vi "401_Sort 2 Column Array By First Column.vi"(1 "Data_Table":string[][](array[string])) -> (0 "Array":string[][](array[string]))   [LabVIEW 2015]
doc: "This vi sorts a two-column array in reference to its first column."
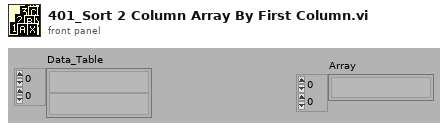
[diagram p1: front panel]
types:
  T1 = cluster{string, string, string, string, string, string, string}[]
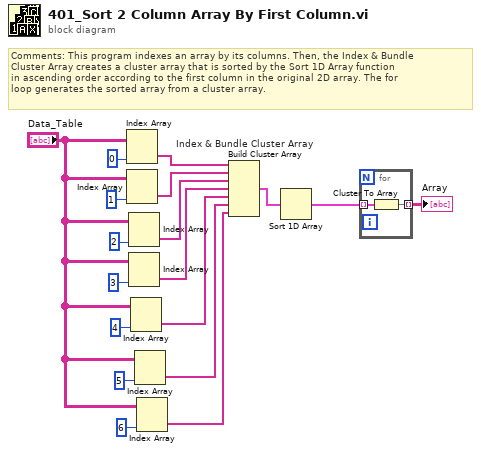
[diagram p0: block diagram]
diagram:
  # "Comments: This program indexes an array by its columns. Then, the Index & Bundle\nCluster Array creates a cluster array that is sorted by the Sort 1D Array function\nin ascending order according to the first column in the original 2D array. The for\nloop generates the sorted array from a cluster array."
  n1 = Index Array(array="Data_Table", index (col)=0) -> (element=w18:string[])  [unwired: 1 in]
  n2 = Index Array(array="Data_Table", index (col)=1) -> (element=w17:string[])  [unwired: 1 in]
  n3 = Index Array(array="Data_Table", index (col)=2) -> (element=w11:string[])  [unwired: 1 in]
  n4 = Index Array(array="Data_Table", index (col)=3) -> (element=w10:string[])  [unwired: 1 in]
  n5 = Index Array(array="Data_Table", index (col)=4) -> (element=w5:string[])  [unwired: 1 in]
  n6 = Index Array(array="Data_Table", index (col)=5) -> (element=w4:string[])  [unwired: 1 in]
  n7 = Index Array(array="Data_Table", index (col)=6) -> (element=w3:string[])  [unwired: 1 in]
  n8 = Build Cluster Array "Index & Bundle Cluster Array"(w18, w17, w11, w10, w5, w4, w3) -> (w2:T1)
  n9 = Sort 1D Array(array=w2) -> (sorted array=w16:T1)
  n10 = for {
    tunnel: w16 -> [w19] mode=indexing
    tunnel: [w20] -> w1 mode=indexing
    n11 = Cluster To Array(cluster=w19) -> (array=w20:string[])
  }
  "Array" <- w1
